vi "Capture_and_read_easy.vi"() -> ()   [LabVIEW 2018]
panel:
  out "Error?":bool
  in  "Capture Range":u32(ring) items=["Auto", "Low", "Medium", "High", "Super", "Ultra"]
  in  "FIBER":u32=1 min=1 max=20 step=1
  out "SATURATION":u32
  out "INTENSITY":u32
  out "HUE":dbl
  in  "VISA resource name":refnum<visa-resource-name>="ASRL34::INSTR"
  # "NOTE: remember plug-in the LED Analyser\ncable before run this VI and to select the\nVISA resource name (port)"
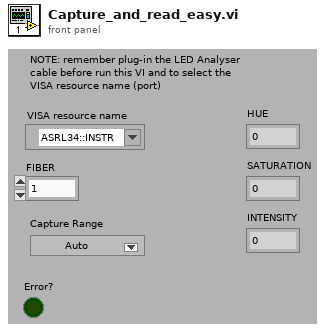
[diagram p1: front panel]
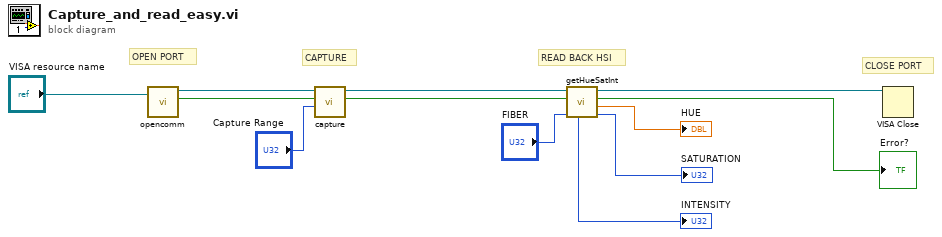
[diagram p0: block diagram]
diagram:
  # "CLOSE PORT"
  # "READ BACK HSI"
  # "CAPTURE"
  # "OPEN PORT"
  n1 = call "opencomm.vi"("VISA resource name"="VISA resource name") -> ("duplicate VISA resource name"=w11:refnum<visa-resource-name>, "Error"=w10:bool)  [unwired: 3 in]
  n2 = call "capture.vi"("Capture Range (0, auto)"="Capture Range", "isPWM (no)"=w10, "VISA resource name"=w11) -> ("Error"=w7:bool, "dup VISA resource name"=w9:refnum<visa-resource-name>)  [unwired: 3 in]
  n3 = call "getHueSatInt.vi"("Fiber Num"="FIBER", "Error"=w7, "VISA resource name"=w9) -> ("Saturation"=→"SATURATION":u32, "Hue"=→"HUE":dbl, "Error"=→"Error?":bool, "dup VISA resource name"=w8:refnum<visa-resource-name>, "Intensity"=→"INTENSITY":u32)  [unwired: 2 in]
  n4 = VISA Close(VISA resource name=w8) -> ()  [unwired: 1 in, 1 out]
